vi "LVCAM Propagate Error.vi"(10 "error in":errorcluster, 11 "Self Actor in":refnum<class "Self Actor.lvclass">) -> (0 "error out":errorcluster)   [LabVIEW 2021, in "LVCAM.lvlib" / "Self Actor.lvclass"]
uses:
  Self Actor.lvclass
  C:/PPLs/LabVIEW-Composed-Actor-Model-LVCAM/LabVIEW-Composed-Actor-Model-LVCAM/LVCAM/LVCAM/LVCAM/LVCAM.lvclass
  Msgs/LVCAM Destroy Self/LVCAM Destroy Self Msg/LVCAM Destroy Self Msg.lvclass
  C:/PPLs/LabVIEW-Composed-Actor-Model-LVCAM/LabVIEW-Composed-Actor-Model-LVCAM/LVCAM/LVCAM/Msg/Msg.lvclass
  Self Msg Send.vi
  C:/PPLs/LabVIEW-Composed-Actor-Model-LVCAM/LabVIEW-Composed-Actor-Model-LVCAM/LVCAM/Msgs/LVCAM Create Nest/LVCAM Create Nest/LVCAM Create Nest.lvclass
  C:/PPLs/LabVIEW-Composed-Actor-Model-LVCAM/LabVIEW-Composed-Actor-Model-LVCAM/LVCAM/Msgs/LVCAM Destroy Self/LVCAM Destroy Self/LVCAM Destroy Self.lvclass
  C:/PPLs/LabVIEW-Composed-Actor-Model-LVCAM/LabVIEW-Composed-Actor-Model-LVCAM/LVCAM/Msgs/LVCAM Nest Destroyed/LVCAM Nest Destroyed/LVCAM Nest Destroyed.lvclass
  C:/PPLs/LabVIEW-Composed-Actor-Model-LVCAM/LabVIEW-Composed-Actor-Model-LVCAM/LVCAM/LVCAM/LVCAM Destroy/LVCAM Destroy.lvclass
  C:/PPLs/LabVIEW-Composed-Actor-Model-LVCAM/LabVIEW-Composed-Actor-Model-LVCAM/LVCAM/LVCAM/LVCAM Create/LVCAM Create.lvclass
  C:/PPLs/LabVIEW-Composed-Actor-Model-LVCAM/LabVIEW-Composed-Actor-Model-LVCAM/LVCAM/LVCAM/LVCAM Msg Receive/LVCAM Msg Receive.lvclass
  C:/PPLs/LabVIEW-Composed-Actor-Model-LVCAM/LabVIEW-Composed-Actor-Model-LVCAM/LVCAM/LVCAM/LVCAM Propagate Error/LVCAM Propagate Error.lvclass
  C:/PPLs/LabVIEW-Composed-Actor-Model-LVCAM/LabVIEW-Composed-Actor-Model-LVCAM/LVCAM/LVCAM/Self Actor/Self Actor.lvclass
  C:/PPLs/LabVIEW-Composed-Actor-Model-LVCAM/LabVIEW-Composed-Actor-Model-LVCAM/LVCAM/Msgs/LVCAM Destroy Self/LVCAM Destroy Self Msg/LVCAM Destroy Self Msg.lvclass
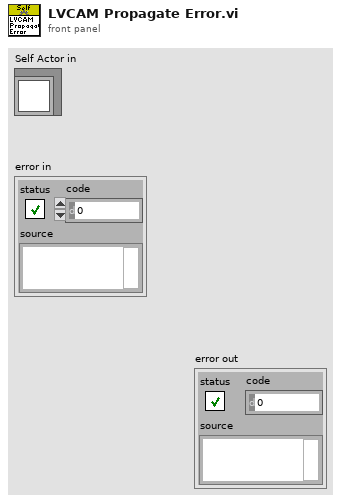
[diagram p1: front panel]
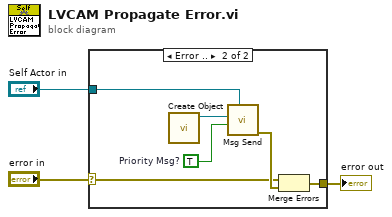
[diagram p0: block diagram]
diagram:
  n1 = case shown="Error .." "error in" {
    selector: "error in" -> [_ w4]
    tunnel: "Self Actor in" -> [_ w7]
    tunnel: [_ w6] -> w1
    frame No Error {
    }
    frame Error {
      w8 = TRUE  # Priority Msg?
      n2 = call "Create Object.vi"() -> ("LVCAM Destroy Self Msg out"=w9:refnum<class "LVCAM Destroy Self Msg.lvclass">)  [unwired: 11 in]
      n3 = call-poly "Msg Send.vi"("Self Actor"=w7, "Priority Msg?"=w8, "Msg"=w9) -> ("error out"=w5:errorcluster)  [unwired: 8 in]
      n4 = Merge Errors(w4, w5) -> (w6:errorcluster)
    }
  }
  "error out" <- w1
